vi "Set Formatter.vi"(8 "error in":errorcluster, 10 "Formatter.lvclass":refnum<class "Formatter.lvclass">, 11 "FileHandler":refnum<class "FileHandler.lvclass">) -> (0 "error out":errorcluster, 3 "FileHandler out":refnum<class "FileHandler.lvclass">)   [LabVIEW 2016, in "hse-logger.lvlib" / "FileHandler.lvclass"]
doc: "Sets the Formatter for this handler to fmt."
uses:
  FileHandler.lvclass
  Formatter/Formatter.lvclass
  FileHandler.lvclass/FileHandler.ctl
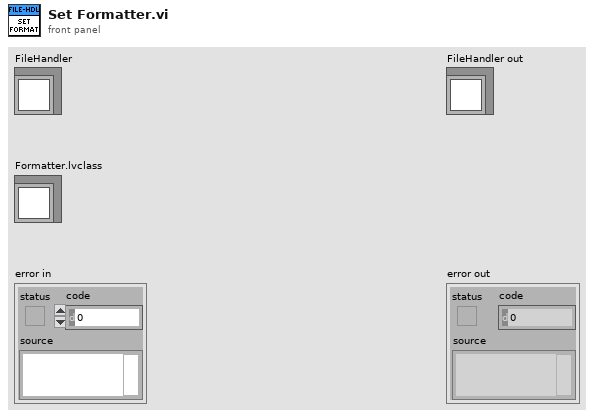
[diagram p1: front panel]
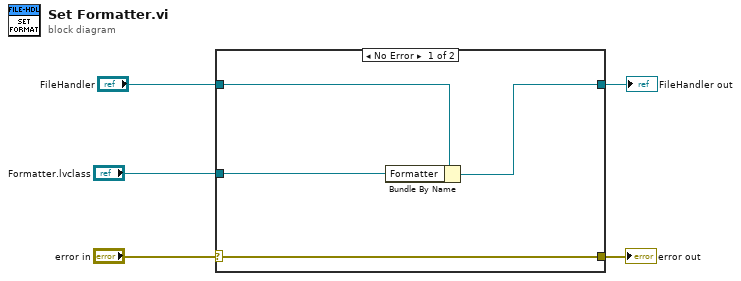
[diagram p0: block diagram]
diagram:
  n1 = case shown="No Error" "error in" {
    selector: "error in" -> [w9 w11]
    tunnel: [w9 w11] -> w4
    tunnel: [w7 w10] -> w1
    tunnel: "FileHandler" -> [w8 w10]
    tunnel: "Formatter.lvclass" -> [w6 _]
    frame No Error {
      n2 = Bundle By Name(cluster=w8, "Formatter"=w6) -> (w7:refnum<class "FileHandler.lvclass">)
    }
    frame Error {
    }
  }
  "error out" <- w4
  "FileHandler out" <- w1
